vi "Create All Message Queues.vi"(8 "error in (no error)":T1 caption="entrée d'erreur (pas d'erreur)", 11 "Stop Event":refnum<user-event>) -> (0 "error out":T1 caption="sortie d'erreur", 3 "Fifo":T2)   [LabVIEW 2020, in "Message Queue.lvlib"]
doc: "Ce VI crée et initialise toutes les files d'attente de messages de l'application. Si votre application requiert plusieurs files d'attente de messages, cliquez sur la constante \"Message Queues\" ci-dessus avec le bouton droit et sélectionnez Ouvrir la déf. de type. Ajoutez les nouvelles files d'attente de messages à la définition de type puis initialisez-les dans ce VI."
uses:
  Message Queue.lvlib
  All Message Queues.ctl
  Message Cluster.ctl
  controls/Ctrl_Ref.ctl
  Enqueue Message (Single).vi
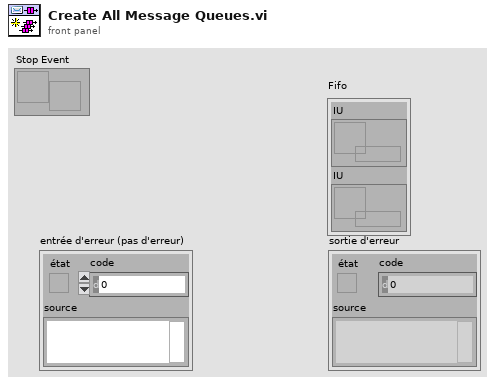
[diagram p1: front panel]
types:
  T1 = cluster{"état":bool, "code":i32, "source":string}
  T2 = typedef "Message Queue.lvlib/All Message Queues.ctl" = cluster{"Conductor":refnum<queue>, "IU":refnum<queue>}
  T3 = typedef "Ctrl_Ref.ctl" = cluster{"Fifo":T2, "Event":cluster{"Stop":refnum<user-event>}}
  T4 = cluster{"[0]":refnum<queue>, "[1]":refnum<queue>}
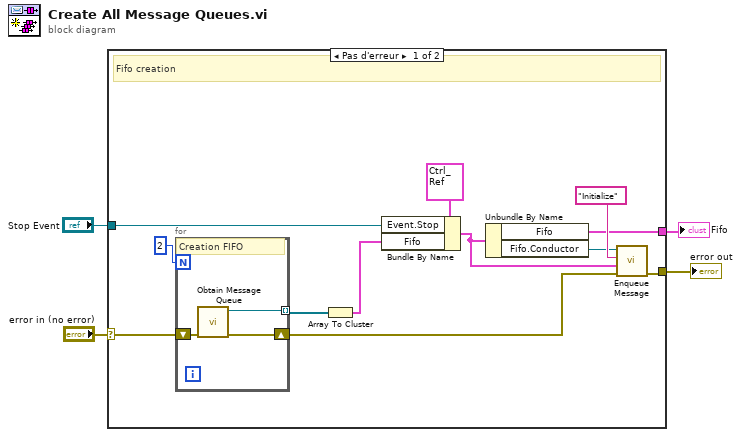
[diagram p0: block diagram]
diagram:
  n1 = case shown="Pas d'erreur" "error in (no error)" {
    selector: "error in (no error)" -> [w16 w20]
    tunnel: [w10 w20] -> w4
    tunnel: [w5 _] -> w2
    tunnel: "Stop Event" -> [w8 _]
    frame No Error {
      # "Fifo creation"
      n2 = for {
        N: 2 -> [_]
        shift-right: [w17] -> w11
        shift-left: w16 -> [w19]
        tunnel: [w18] -> w14 mode=indexing
        # "Creation FIFO"
        n3 = call "Obtain Message Queue.vi"("error in (no error)"=w19) -> ("error out"=w17:T1, "File d'attente de messages"=w18:refnum<queue>)  [unwired: 9 in]
      }
      n4 = Array To Cluster(array=w14) -> (cluster=w7:T4)
      n5 = Bundle By Name(cluster=T3 {"Fifo"={"Conductor"=refnum, "IU"=refnum}, "Event"={"Stop"=refnum}} ("Ref"), "Event.Stop"=w8, "Fifo"=w7) -> (w6:T3)
      n6 = Unbundle By Name(w6) -> ("Fifo"=w5:T2, "Fifo.Conductor"=w12:refnum<queue>)
      n7 = call-poly "Enqueue Message.vi"("error in (no error)"=w11, "Données de message"=w6, "Message"="Initialize", "File d'attente de messages"=w12) -> ("error out"=w10:T1)  [unwired: 6 in, 1 out]
    }
    frame Error {
    }
  }
  "Fifo" <- w2
  "error out" <- w4
